vi "FTW-Endpoint-CreateReplier.vi"(0 "FTW-Endpoint In":refnum<class "FTW-Endpoint.lvclass">, 11 "error in":errorcluster) -> (4 "FTW-Endpoint Out":refnum<class "FTW-Endpoint.lvclass">, 15 "error out":errorcluster)   [LabVIEW 2013, in "FTW-Endpoint.lvclass"]
uses:
  FTW-Endpoint.lvclass
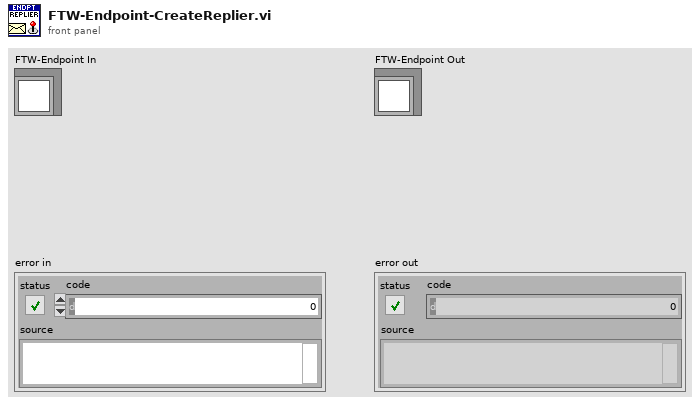
[diagram p1: front panel]
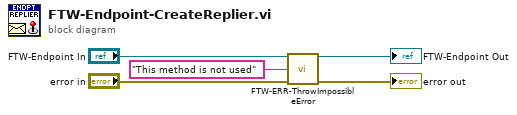
[diagram p0: block diagram]
diagram:
  n1 = call "FTW-ERR-ThrowImpossibleError.vi"("Reason this error should never happen"="This method is not used", "error in"="error in") -> ("error out"=→"error out":errorcluster)  [unwired: 13 in]
  "FTW-Endpoint Out" <- "FTW-Endpoint In"
